vi "GEOM_GUI_GetDetInfo.vi"(9 "index":i32, 10 "fpa info in":string[][](array[string])) -> (1 "col headers":string[](array[string]), 2 "item names":string[][](array[string]))   [LabVIEW 2016]
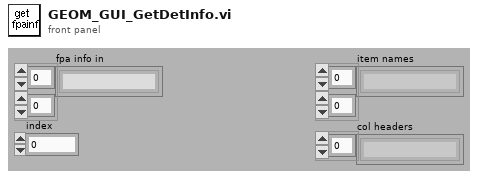
[diagram p1: front panel]
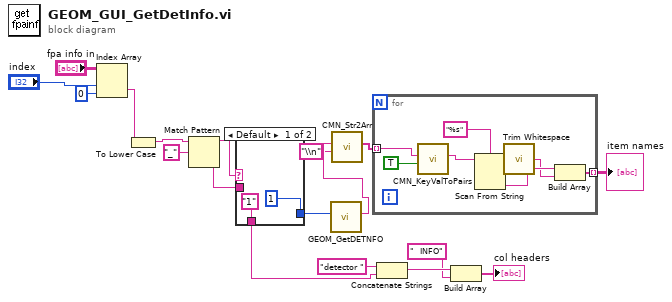
[diagram p0: block diagram]
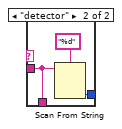
[diagram p2: hidden frame]
diagram:
  n1 = Index Array(array="fpa info in", index (row)="index", index (col)=0 ("disabled index (col)")) -> (element=w17:string)
  n2 = To Lower Case(string=w17) -> (all lower case string=w2:string)
  n3 = Match Pattern(string=w2, regular expression="_") -> (before substring=w7:string, after substring=w15:string)  [unwired: 3 out]
  n4 = case shown="Default" w7 {
    tunnel: w15 -> [_ w21]
    tunnel: [1 w22] -> w14
    tunnel: ["1" w21] -> w6
    frame Default {
    }
    frame "detector" {
      n5 = Scan From String(format string="%d", input string=w21) -> (output 1=w22:i32)  [unwired: 2 in, 4 out]
    }
  }
  n6 = call "GEOM_GetDETNFO.vi"("detnum"=w14) -> ("info"=w13:string)  [unwired: 1 in, 9 out]
  n7 = call "CMN_Str2Arr.vi"("separator"="\\n", "string in"=w13) -> ("Array out"=w12:string[])  [unwired: 2 in, 7 out]
  n8 = for {
    tunnel: w12 -> [w31] mode=indexing
    tunnel: [w24] -> w4 mode=indexing
    n9 = call "CMN_KeyValToPairs.vi"("replace all? (F)"=TRUE, "key=value pairs"=w31) -> ("arguments out"=w29:string)  [unwired: 9 out]
    n10 = Scan From String(format string="%s", input string=w29) -> (remaining string=w26:string, output 1=w27:string)  [unwired: 2 in, 3 out]
    n11 = call <vilib>:"Trim Whitespace.vi"("string"=w26) -> ("trimmed string"=w25:string)  [unwired: 1 in]
    n12 = Build Array(w27, w25) -> (w24:string[])
  }
  "item names" <- w4
  n13 = Concatenate Strings("detector " ("string"), w6) -> (w9:string)
  n14 = Build Array(w9, "  INFO" ("element")) -> (→"col headers":string[])
